vi "formatReading.vi"(8 "error in (no error)":errorcluster, 11 "Electrometer in":refnum<class "Electrometer.lvclass">) -> (0 "error out":errorcluster, 3 "Electrometer out":refnum<class "Electrometer.lvclass">)   [LabVIEW 2016, in "Electrometer.lvclass"]
uses:
  Electrometer.lvclass
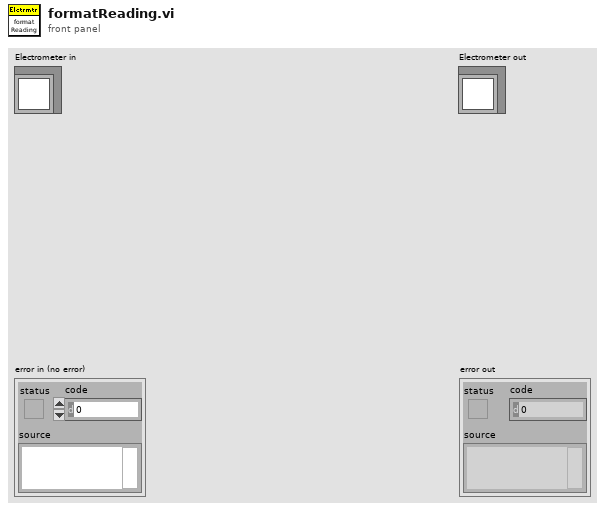
[diagram p1: front panel]
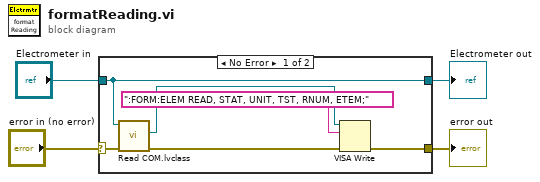
[diagram p0: block diagram]
diagram:
  n1 = case shown="No Error" "error in (no error)" {
    selector: "error in (no error)" -> [w9 w12]
    tunnel: [w5 w12] -> w3
    tunnel: [w8 w11] -> w1
    tunnel: "Electrometer in" -> [w8 w11]
    frame No Error {
      n2 = call "Read COM.lvclass.vi"("error in (no error)"=w9, "Electrometer in"=w8) -> ("error out"=w7:errorcluster, "VISA"=w10:refnum<visa-resource-name>)  [unwired: 7 in, 1 out]
      n3 = VISA Write(VISA resource name=w10, write buffer=":FORM:ELEM READ, STAT, UNIT, TST, RNUM, ETEM;", error in (no error)=w7) -> (error out=w5:errorcluster)  [unwired: 2 out]
    }
    frame Error {
    }
  }
  "error out" <- w3
  "Electrometer out" <- w1
